vi "Check SysDef for VCOM Signal.vi"(8 "error in (no error)":errorcluster, 10 "VCOM Signal Map In":map{string, T1}(c390), 11 "System Definition File Path":path=path "C:/Users/Nick/Desktop/VCOM Config System Definition Utility/VeriStand Example Project/Example Project/Example Project.nivssdf") -> (0 "error out":errorcluster, 3 "Signals Not Found in new VCOM Config":string[](array[string]))   [LabVIEW 2025]
uses:
  <vilib>/Vehicle Communication Toolkit/TypDefs/RBS Signal.ctl
  NationalInstruments.VeriStand.SystemDefinitionAPI
  <vilib>/NI/NI VeriStand Advanced SysDef API/_SubVIs/SysDef.Search.GUIDs.vi
  NationalInstruments.VeriStand.SystemStorage
  <vilib>/NI/NI VeriStand Advanced SysDef API/SysDef API/Advanced System Definition.lvlib
  <vilib>/Vehicle Communication Toolkit/Vehicle Communication Toolkit.lvlib
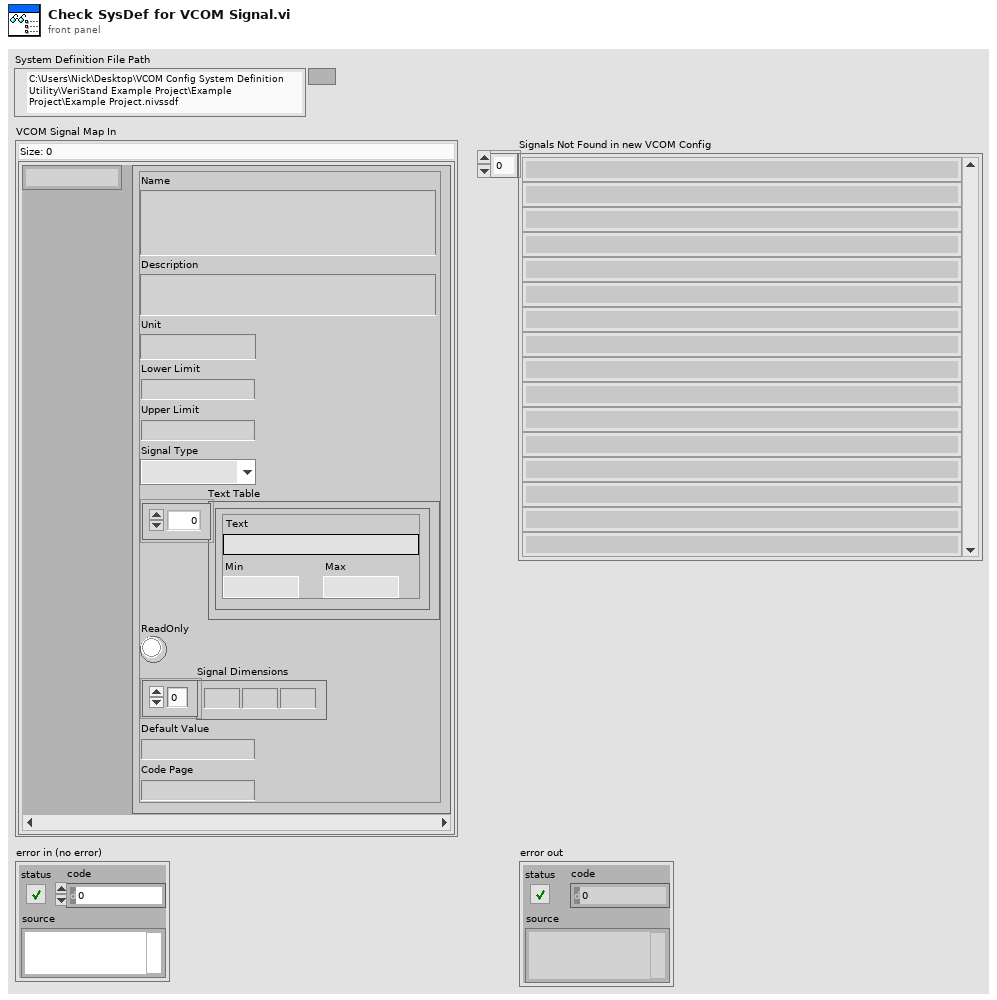
[diagram p1: front panel]
types:
  T1 = typedef "Vehicle Communication Toolkit.lvlib/RBS Signal.ctl" = cluster{"Name":string, "Description":string, "Unit":string, "Lower Limit":dbl, "Upper Limit":dbl, "Signal Type":enum32{"RE_BOOL", "RE_UINT8", "RE_INT8", "RE_UINT16", "RE_INT16", "RE_UINT32", "RE_INT32", "RE_UINT64", "RE_INT64", "RE_FLOAT32", "RE_FLOAT64", "RE_TEXT"}, "Text Table":cluster{"Text":string, "Min":dbl, "Max":dbl}[], "ReadOnly":bool, "Signal Dimensions":u32[], "Default Value":dbl, "Code Page":u32}
  T2 = typedef "Custom Device API.lvlib/Custom Device Pointer.ctl" = refnum<k24>
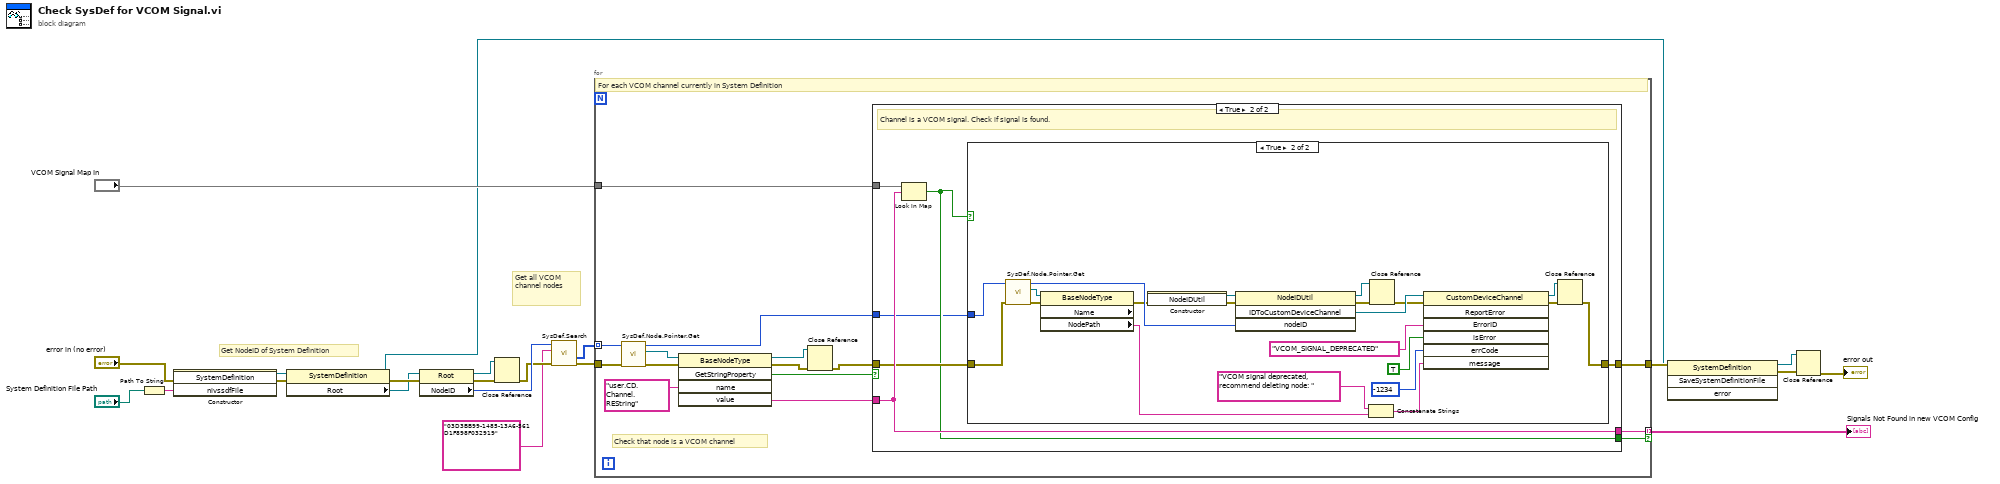
[diagram p0: block diagram]
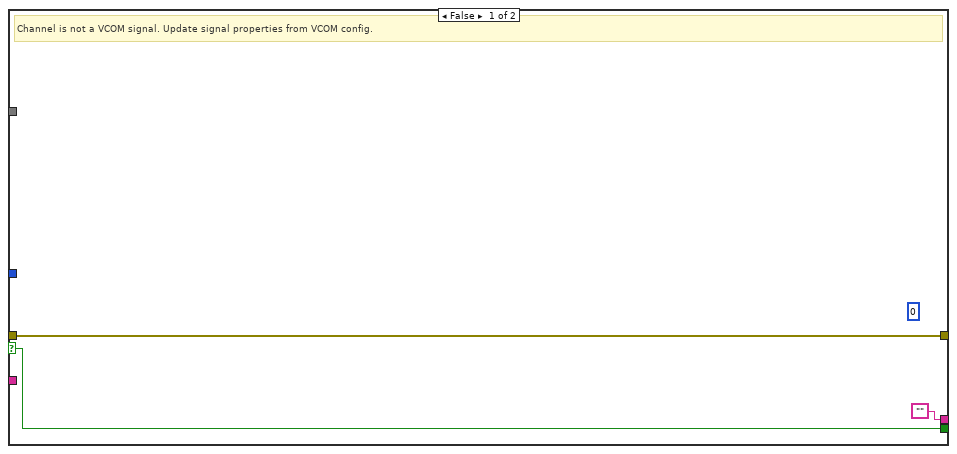
[diagram p2: hidden frame]
diagram:
  # "Get all VCOM channel nodes"
  # "Get NodeID of System Definition"
  n1 = Path To String(path="System Definition File Path") -> (string=w19:string)
  n2 = constructor class="SystemDefinition"(error in="error in (no error)", "nivssdfFile"=w19) -> (reference out=w17:refnum<k24>, error out=w18:errorcluster)  [unwired: 2 in, 2 out]
  n3 = property class="SystemDefinition"(reference=w17, error in=w18) -> (reference out=w4:refnum<k24>, error out=w15:errorcluster, "Root"=w7:refnum<k24>)
  n4 = property class="Root"(reference=w7, error in=w15) -> (reference out=w12:refnum<k24>, error out=w13:errorcluster, "NodeID"=w14:u64)
  n5 = Close Reference(reference=w12, error in (no error)=w13) -> (error out=w11:errorcluster)
  n6 = call-poly <vilib>:"SysDef.Search.vi"("error in (no error)"=w11, "GUID"="03D3BB99-1485-13A6-561D1F898F032919", "nodeID"=w14) -> ("error out"=w21:errorcluster, "Values Out"=w20:u64[])  [unwired: 5 in, 2 out]
  n7 = for {
    tunnel: w20 -> [w30] mode=indexing
    tunnel: "VCOM Signal Map In" -> [w32]
    tunnel: w21 -> [w34]
    tunnel: [w28] -> w5
    tunnel: [w26] -> w6 mode=indexing if=w25
    # "Check that node is a VCOM channel"
    # "For each VCOM channel currently in System Definition"
    n8 = call <vilib>:"SysDef.Node.Pointer.Get.vi"("error in (no error)"=w34, "nodeID"=w30) -> ("error out"=w33:errorcluster, "Node Pointer"=w36:T2, "nodeID out"=w29:u64)  [unwired: 6 in, 1 out]
    n9 = invoke class="BaseNodeType" method="GetStringProperty"(reference=w36, error in=w33, "name"="user.CD.Channel.REString") -> (reference out=w23:T2, error out=w24:errorcluster, "GetStringProperty"=w27:bool, "value"=w31:string)  [unwired: 2 in, 1 out]
    n10 = Close Reference(reference=w23, error in (no error)=w24) -> (error out=w22:errorcluster)
    n11 = case shown="True" w27 {
      selector: w27 -> [w38 _]
      tunnel: w32 -> [_ w45]
      tunnel: w31 -> [_ w44]
      tunnel: w22 -> [w39 w43]
      tunnel: w29 -> [_ w41]
      tunnel: [w39 w40] -> w28
      tunnel: ["" w44] -> w26
      tunnel: [w38 w42] -> w25
      frame False {
        (unwired) u64 0 ("nodeID out")
        # "Channel is not a VCOM signal. Update signal properties from VCOM config."
      }
      frame True {
        # "Channel is a VCOM signal. Check if signal is found."
        n12 = Look In Map(map=w45, key=w44) -> (key not found?=w42:bool)  [unwired: 1 in, 1 out]
        n13 = case shown="True" w42 {
          tunnel: w43 -> [w46 w67]
          tunnel: w41 -> [_ w66]
          tunnel: [w46 w65] -> w40
          frame False {
          }
          frame True {
            n14 = call <vilib>:"SysDef.Node.Pointer.Get.vi"("error in (no error)"=w67, "nodeID"=w66) -> ("error out"=w61:errorcluster, "Node Pointer"=w62:T2, "nodeID out"=w60:u64)  [unwired: 6 in, 1 out]
            n15 = property class="BaseNodeType" props=["Name", "NodePath"](reference=w62, error in=w61) -> (error out=w54:errorcluster, "NodePath"=w48:string)  [unwired: 2 out]
            n16 = constructor class="NodeIDUtil"(error in=w54) -> (reference out=w53:refnum<k24>, error out=w55:errorcluster)  [unwired: 2 in, 1 out]
            n17 = invoke class="NodeIDUtil" method="IDToCustomDeviceChannel"(reference=w53, error in=w55, "nodeID"=w60) -> (reference out=w52:refnum<k24>, error out=w51:errorcluster, "IDToCustomDeviceChannel"=w56:refnum<k24>)  [unwired: 1 in, 1 out]
            n18 = Concatenate Strings("VCOM signal deprecated, recommend deleting node: " ("ErrorID"), w48) -> (w47:string)
            n19 = Close Reference(reference=w52, error in (no error)=w51) -> (error out=w50:errorcluster)
            n20 = invoke class="CustomDeviceChannel" method="ReportError"(reference=w56, error in=w50, "ErrorID"="VCOM_SIGNAL_DEPRECATED", "isError"=TRUE, "errCode"=-1234, "message"=w47) -> (reference out=w63:refnum<k24>, error out=w64:errorcluster)  [unwired: 1 in, 5 out]
            n21 = Close Reference(reference=w63, error in (no error)=w64) -> (error out=w65:errorcluster)
          }
        }
      }
    }
  }
  "Signals Not Found in new VCOM Config" <- w6
  n22 = invoke class="SystemDefinition" method="SaveSystemDefinitionFile"(reference=w4, error in=w5) -> (reference out=w2:refnum<k24>, error out=w3:errorcluster)  [unwired: 2 in, 2 out]
  n23 = Close Reference(reference=w2, error in (no error)=w3) -> (error out=→"error out":errorcluster)
